vi "Acquire Once.vi"(8 "error in (no error)":errorcluster caption="错误输入（无错误）", 11 "Settings":T1={"Hardware Configuration"={"电压读取设置"={"DAQmx Channel"="", "Max Input"=0.0, "Min Input"=0.0, "Sample Rate"=0.0, "Sample Number"=0, "DAQmx Task"="", "device in"=""}, "角度传感器设置"={"counter"="Dev1/ctr0", "units"=10146, "分辨率"=0, "初始角度"=0.0, "DecodingType"=10092, "A相端口"="/Dev1/PFI8", "B相端口"="/Dev1/PFI8", "task in"=""}}, "Logging Configuration"={"Log File Base Path"=path "", "电压传感器转换率"=[], "电压传感器本底"=[]}, "电机设置"={"counter"="Dev1/ctr0", "方向端口"="", "当前方向"=FALSE, "频率"=0.0, "DAQmx Task"=""}, "啮合测试电机转动逻辑"={"反转判断条件1"={"传感器序号"=0, "条件"=enum."小于", "值"=0.0, "条件判断时间间隔"=0, "反转等待时长"=0}, "停止判断条件1"={"角度传感器序号"=0, "正转/反转"=enum."正转", "反转次数"=0, "停止角度"=0.0, "停止角度误差范围"=0.0}}, "功能测试电机转动逻辑"={"反转判断条件1"={"传感器序号"=0, "条件"=enum."小于", "值"=0.0, "条件判断时间间隔"=0, "反转等待时长"=0}, "停止判断条件1"={"角度传感器序号"=0, "正转/反转"=enum."正转", "反转次数"=0, "停止角度"=0.0, "停止角度误差范围"=0.0}}, "力提特性电机转动逻辑"={"反转判断条件1"={"传感器序号"=0, "条件"=enum."小于", "值"=0.0, "条件判断时间间隔"=0, "反转等待时长"=0}, "停止判断条件1"={"角度传感器序号"=0, "正转/反转"=enum."正转", "反转次数"=0, "停止角度"=0.0, "停止角度误差范围"=0.0}}, "内泄漏测试电机转动逻辑"={"反转判断条件1"={"传感器序号"=0, "条件"=enum."小于", "值"=0.0, "条件判断时间间隔"=0, "反转等待时长"=0}, "停止判断条件1"={"角度传感器序号"=0, "正转/反转"=enum."正转", "反转次数"=0, "停止角度"=0.0, "停止角度误差范围"=0.0}}, "PLC设置"={"端口选择"="COM3", "波特率"=9600, "校检"=2, "数据位"=7}, "PLC动作指令集"={"PLC动作指令1"={"变量类型"=2, "PLC地址"="0", "16位/32位"=0, "写入数据(写入时有效)"=""}, "PLC动作指令2"={"变量类型"=2, "PLC地址"="0", "16位/32位"=0, "写入数据(写入时有效)"=""}, "PLC动作指令3"={"变量类型"=2, "PLC地址"="0", "16位/32位"=0, "写入数据(写入时有效)"=""}}} caption="设置" {"PLC动作指令集"."PLC动作指令3"."16位/32位" items=["16bit", "32bit"]; "PLC动作指令集"."PLC动作指令3"."变量类型" items=["X", "Y", "M", "D"]; "PLC动作指令集"."PLC动作指令2"."16位/32位" items=["16bit", "32bit"]; "PLC动作指令集"."PLC动作指令2"."变量类型" items=["X", "Y", "M", "D"]; "PLC动作指令集"."PLC动作指令1"."16位/32位" items=["16bit", "32bit"]; "PLC动作指令集"."PLC动作指令1"."变量类型" items=["X", "Y", "M", "D"]; "PLC设置"."数据位" items=["7"=7, "8"=8]; "PLC设置"."校检" items=["无", "偶", "奇"]; "PLC设置"."波特率" items=["9600"=9600, "19200"=19200, "115200"=115200]; "Hardware Configuration"."角度传感器设置"."DecodingType" items=["X1"=10090, "X2"=10091, "X4"=10092, "Two Pulse Counting"=10313]; "Hardware Configuration"."角度传感器设置"."units" items=["Degrees"=10146, "Radians"=10273, "Ticks"=10304, "From Custom Scale"=10065]}) -> (0 "error out":errorcluster caption="错误输出", 2 "信号数据":dbl[][](array[numeric]), 3 "Settings 2":T1={"Hardware Configuration"={"电压读取设置"={"DAQmx Channel"="", "Max Input"=0.0, "Min Input"=0.0, "Sample Rate"=0.0, "Sample Number"=0, "DAQmx Task"="", "device in"=""}, "角度传感器设置"={"counter"="Dev1/ctr0", "units"=10146, "分辨率"=0, "初始角度"=0.0, "DecodingType"=10092, "A相端口"="/Dev1/PFI8", "B相端口"="/Dev1/PFI8", "task in"=""}}, "Logging Configuration"={"Log File Base Path"=path "", "电压传感器转换率"=[], "电压传感器本底"=[]}, "电机设置"={"counter"="Dev1/ctr0", "方向端口"="", "当前方向"=FALSE, "频率"=0.0, "DAQmx Task"=""}, "啮合测试电机转动逻辑"={"反转判断条件1"={"传感器序号"=0, "条件"=enum."小于", "值"=0.0, "条件判断时间间隔"=0, "反转等待时长"=0}, "停止判断条件1"={"角度传感器序号"=0, "正转/反转"=enum."正转", "反转次数"=0, "停止角度"=0.0, "停止角度误差范围"=0.0}}, "功能测试电机转动逻辑"={"反转判断条件1"={"传感器序号"=0, "条件"=enum."小于", "值"=0.0, "条件判断时间间隔"=0, "反转等待时长"=0}, "停止判断条件1"={"角度传感器序号"=0, "正转/反转"=enum."正转", "反转次数"=0, "停止角度"=0.0, "停止角度误差范围"=0.0}}, "力提特性电机转动逻辑"={"反转判断条件1"={"传感器序号"=0, "条件"=enum."小于", "值"=0.0, "条件判断时间间隔"=0, "反转等待时长"=0}, "停止判断条件1"={"角度传感器序号"=0, "正转/反转"=enum."正转", "反转次数"=0, "停止角度"=0.0, "停止角度误差范围"=0.0}}, "内泄漏测试电机转动逻辑"={"反转判断条件1"={"传感器序号"=0, "条件"=enum."小于", "值"=0.0, "条件判断时间间隔"=0, "反转等待时长"=0}, "停止判断条件1"={"角度传感器序号"=0, "正转/反转"=enum."正转", "反转次数"=0, "停止角度"=0.0, "停止角度误差范围"=0.0}}, "PLC设置"={"端口选择"="COM3", "波特率"=9600, "校检"=2, "数据位"=7}, "PLC动作指令集"={"PLC动作指令1"={"变量类型"=2, "PLC地址"="0", "16位/32位"=0, "写入数据(写入时有效)"=""}, "PLC动作指令2"={"变量类型"=2, "PLC地址"="0", "16位/32位"=0, "写入数据(写入时有效)"=""}, "PLC动作指令3"={"变量类型"=2, "PLC地址"="0", "16位/32位"=0, "写入数据(写入时有效)"=""}}} caption="Settings" {"PLC动作指令集"."PLC动作指令3"."16位/32位" items=["16bit", "32bit"]; "PLC动作指令集"."PLC动作指令3"."变量类型" items=["X", "Y", "M", "D"]; "PLC动作指令集"."PLC动作指令2"."16位/32位" items=["16bit", "32bit"]; "PLC动作指令集"."PLC动作指令2"."变量类型" items=["X", "Y", "M", "D"]; "PLC动作指令集"."PLC动作指令1"."16位/32位" items=["16bit", "32bit"]; "PLC动作指令集"."PLC动作指令1"."变量类型" items=["X", "Y", "M", "D"]; "PLC设置"."数据位" items=["7"=7, "8"=8]; "PLC设置"."校检" items=["无", "偶", "奇"]; "PLC设置"."波特率" items=["9600"=9600, "19200"=19200, "115200"=115200]; "Hardware Configuration"."角度传感器设置"."DecodingType" items=["X1"=10090, "X2"=10091, "X4"=10092, "Two Pulse Counting"=10313]; "Hardware Configuration"."角度传感器设置"."units" items=["Degrees"=10146, "Radians"=10273, "Ticks"=10304, "From Custom Scale"=10065]})   [LabVIEW 2015, in "Acquisition.lvlib"]
doc: "执行采集。替换程序框图的内容，添加对采集硬件的调用。"
uses:
  Acquisition.lvlib
  Settings/Settings.ctl
  Hardware Configuration.ctl
  Logging/Logging Configuration.ctl
  Motor Control/Hardware Configuration.ctl
  <vilib>/DAQmx/read.llb/DAQmx Read (Analog 2D DBL NChan NSamp).vi
  <vilib>/DAQmx/miscellaneous.llb/DAQmx Fill In Error Info.vi
  <resource>/objmgr/daqmx.rc
  Logging/Logging.lvlib
  Motor Control/Motor Control.lvlib
  Settings/Settings.lvlib
  PLC/PLC.lvlib
panel:
  # "1、扭矩\n\n2、油压\n\n3、左推力\n\n4、右推力\n\n5、流量\n\n6、位移量"
  # "1、扭矩\n\n2、油压\n\n3、左推力\n\n4、右推力\n\n5、流量\n\n6、位移量"
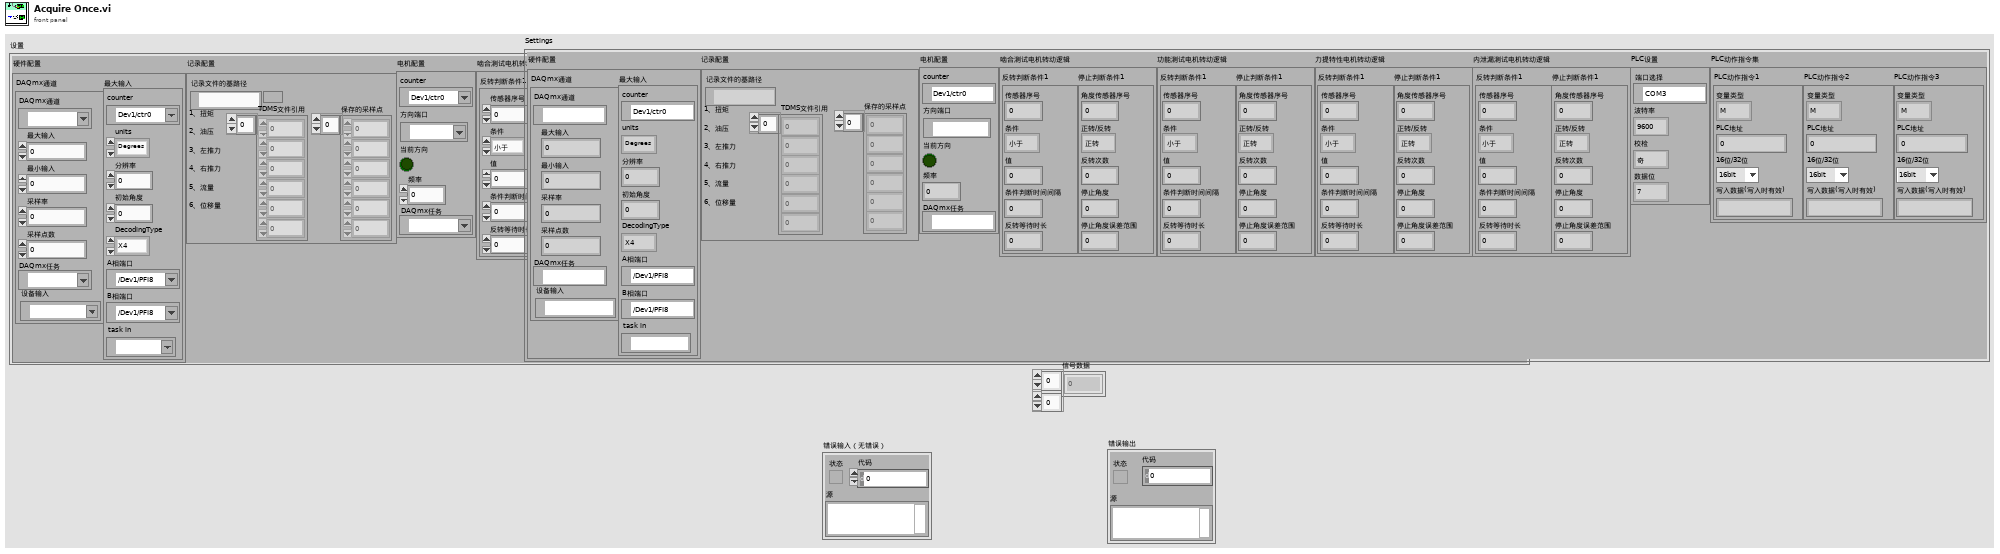
[diagram p1: front panel]
types:
  T1 = typedef "Settings.lvlib/Settings.ctl" = cluster{"Hardware Configuration":T2, "Logging Configuration":T3, "电机设置":T4, "啮合测试电机转动逻辑":T5, "功能测试电机转动逻辑":T5, "力提特性电机转动逻辑":T5, "内泄漏测试电机转动逻辑":T5, "PLC设置":T8, "PLC动作指令集":T9}
  T2 = typedef "Acquisition.lvlib/Hardware Configuration.ctl" = cluster{"电压读取设置":cluster{"DAQmx Channel":tag, "Max Input":dbl, "Min Input":dbl, "Sample Rate":dbl, "Sample Number":i32, "DAQmx Task":refnum<k21>, "device in":tag}, "角度传感器设置":cluster{"counter":tag, "units":i32, "分辨率":i32, "初始角度":dbl, "DecodingType":i32, "A相端口":tag, "B相端口":tag, "task in":refnum<k21>}}
  T3 = typedef "Logging.lvlib/Logging Configuration.ctl" = cluster{"Log File Base Path":path, "电压传感器转换率":dbl[], "电压传感器本底":dbl[]}
  T4 = typedef "Motor Control.lvlib/Hardware Configuration.ctl" = cluster{"counter":tag, "方向端口":tag, "当前方向":bool, "频率":dbl, "DAQmx Task":refnum<k21>}
  T5 = typedef "Motor Control.lvlib/电机转动逻辑1.ctl" = cluster{"反转判断条件1":T6, "停止判断条件1":T7}
  T6 = typedef "Motor Control.lvlib/反转判断条件1.ctl" = cluster{"传感器序号":i32, "条件":enum16{"小于", "大于", "等于"}, "值":dbl, "条件判断时间间隔":i32, "反转等待时长":i32}
  T7 = typedef "Motor Control.lvlib/停止判断条件1.ctl" = cluster{"角度传感器序号":i32, "正转/反转":enum16{"正转", "反转"}, "反转次数":i32, "停止角度":dbl, "停止角度误差范围":dbl}
  T8 = typedef "PLC.lvlib/PLC设置.ctl" = cluster{"端口选择":refnum<visa-resource-name>, "波特率":u32, "校检":u32, "数据位":u32}
  T9 = typedef "PLC.lvlib/PLC动作指令集.ctl" = cluster{"PLC动作指令1":T10, "PLC动作指令2":T10, "PLC动作指令3":T10}
  T10 = typedef "PLC.lvlib/PLC指令.ctl" = cluster{"变量类型":u32, "PLC地址":string, "16位/32位":u32, "写入数据(写入时有效)":string}
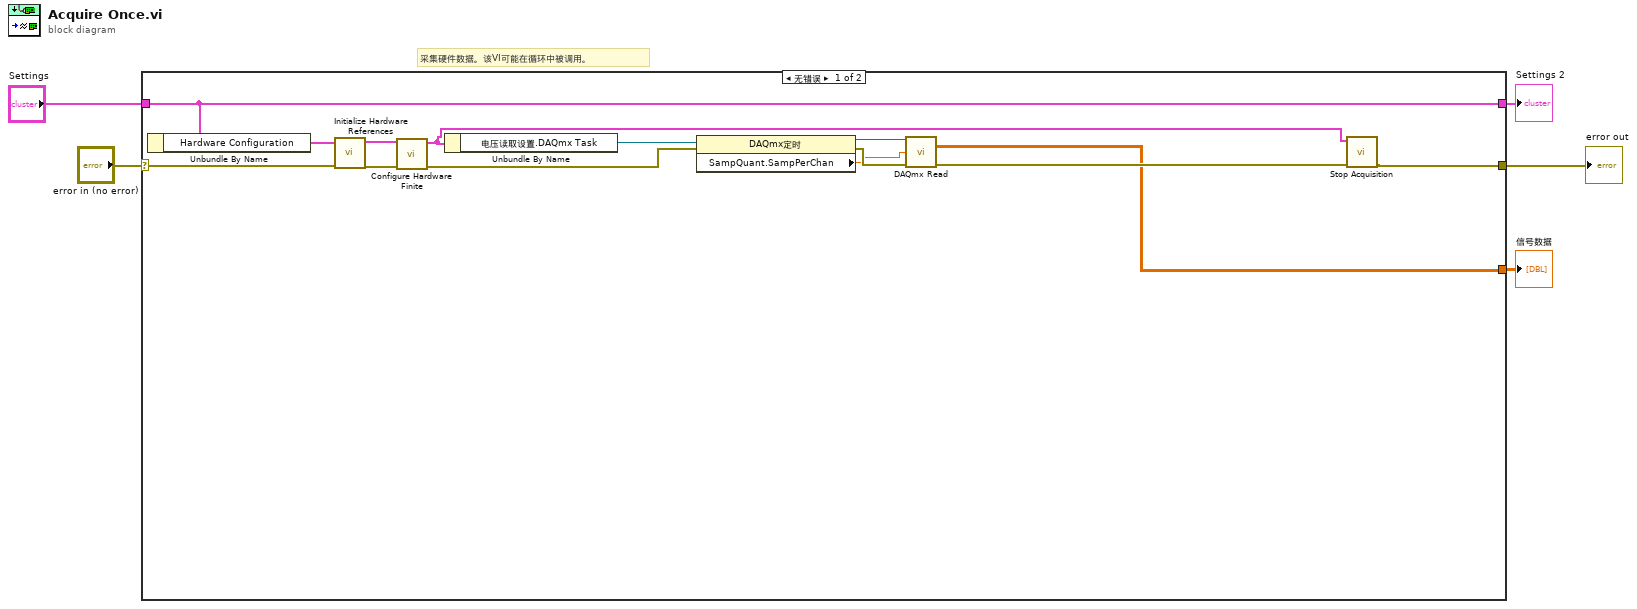
[diagram p0: block diagram]
diagram:
  # "采集硬件数据。该VI可能在循环中被调用。"
  n1 = case shown="无错误" "error in (no error)" {
    selector: "error in (no error)" -> [w19 w20]
    tunnel: [w10 w20] -> w4
    tunnel: "Settings" -> [w7 w21]
    tunnel: [w7 w21] -> w2
    tunnel: [w6 _] -> w1
    frame No Error {
      n2 = Unbundle By Name(w7) -> ("Hardware Configuration"=w14:T2)
      n3 = call "Initialize Hardware References.vi"("error in (no error)"=w19, "Hardware Resources in"=w14) -> ("error out"=w17:errorcluster, "Hardware Resources out"=w18:T2)  [unwired: 8 in]
      n4 = call "Configure Hardware Finite.vi"("error in (no error)"=w17, "Hardware Resources in"=w18) -> ("error out"=w15:errorcluster, "Hardware Resources out"=w8:T2)  [unwired: 8 in]
      n5 = Unbundle By Name(w8) -> ("电压读取设置.DAQmx Task"=w16:refnum<k21>)
      n6 = property class="DAQmx定时"(reference=w16, error in=w15) -> (reference out=w13:refnum<k21>, error out=w12:errorcluster, "SampQuant.SampPerChan"=w11:dbl)
      n7 = call-poly <vilib>:"DAQmx Read.vi"("task/channels in"=w13, "number of samples per channel"=w11, "error in"=w12) -> ("data"=w6:dbl[][], "error out"=w9:errorcluster)  [unwired: 10 in, 1 out]
      n8 = call "Stop Acquisition.vi"("error in (no error)"=w9, "Hardware Resources in"=w8) -> ("error out"=w10:errorcluster)  [unwired: 9 in]
    }
    frame Error {
    }
  }
  "error out" <- w4
  "Settings 2" <- w2
  "信号数据" <- w1
